vi "enablePWM.vi"(7 "targetTorque":i16, 8 "error in (no error)":errorcluster, 10 "targetVelocity":i32, 11 "MotorController in":refnum<class "MotorController.lvclass">) -> (0 "error out":errorcluster, 3 "MotorController out":refnum<class "MotorController.lvclass">)   [LabVIEW 2017, in "MotorController.lvclass"]
uses:
  MotorController.lvclass
  <vilib>/CANopenLib/CANOPEN.llb/CANopen Convert To Data [U16].vi
  <vilib>/CANopenLib/CANOPEN.llb/CANopen Convert To Data [I32].vi
  <vilib>/CANopenLib/CANOPEN.llb/CANopen Convert To Data [I16].vi
panel:
  in  "PDOChannel":u8(ring) items=["PDO 1", "PDO 2", "PDO 3", "PDO 4"]
  in  "CANopen data in":u8[](array[numeric])=[0, 0, 0, 0, 0, 0, 0, 0] format="%.0x"
  out "interface object out":refnum<k20>
  in  "interface object in":refnum<k20>
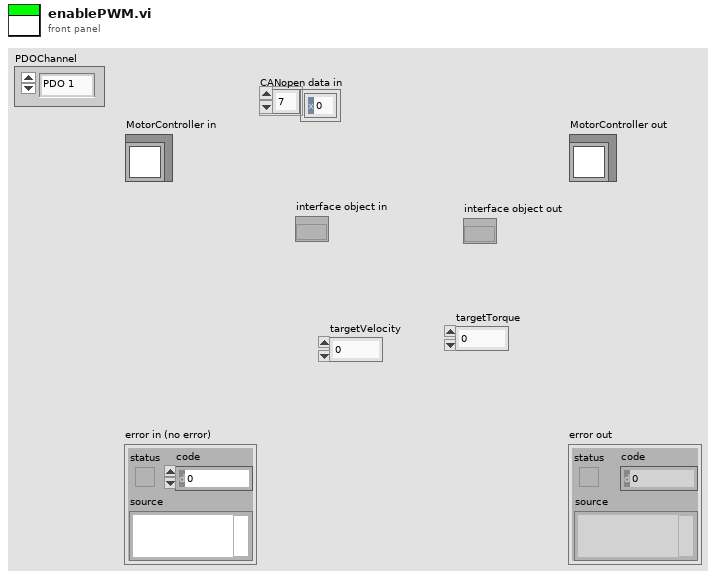
[diagram p1: front panel]
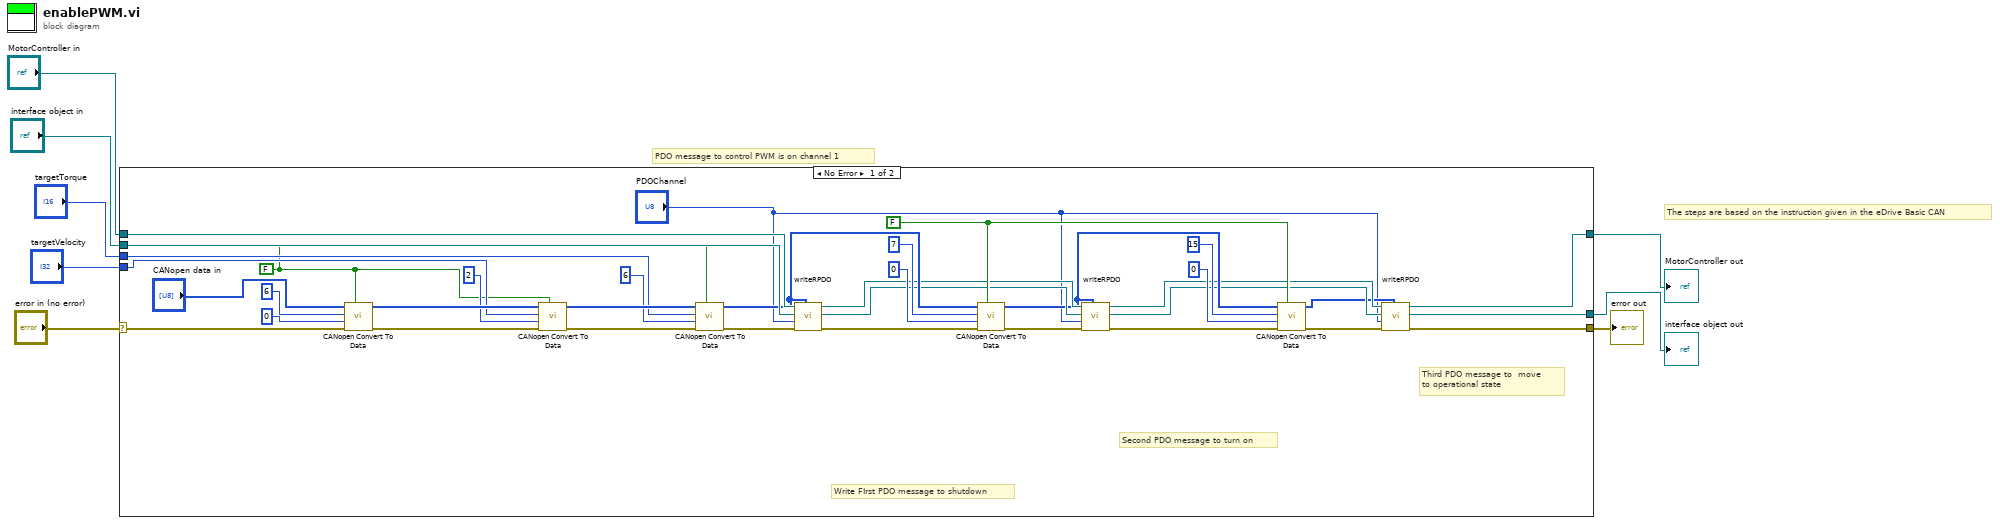
[diagram p0: block diagram]
diagram:
  # "The steps are based on the instruction given in the eDrive Basic CAN"
  # "PDO message to control PWM is on channel 1"
  n1 = case shown="No Error" "error in (no error)" {
    selector: "error in (no error)" -> [w40 w47]
    tunnel: [w10 w47] -> w7
    tunnel: [w11 w46] -> w5
    tunnel: "MotorController in" -> [w44 w46]
    tunnel: "interface object in" -> [w43 w45]
    tunnel: "targetTorque" -> [w32 _]
    tunnel: "targetVelocity" -> [w36 _]
    tunnel: [w12 w45] -> w1
    frame No Error {
      w25 = FALSE ("trim")
      w30 = FALSE ("trim")
      # "Third PDO message to  move \nto operational state"
      # "Second PDO message to turn on"
      # "Write FIrst PDO message to shutdown"
      n2 = call-poly <vilib>:"CANopen Convert To Data.vi"("trim"=w30, "error in (no error)"=w40, "offset (0)"=u32 0, "unsigned 16-bit integer"=u16 6 ("element"), "CANopen data in"="CANopen data in") -> ("error out"=w38:errorcluster, "CANopen data out"=w37:u8[])  [unwired: 5 in]
      n3 = call-poly <vilib>:"CANopen Convert To Data.vi"("trim"=w30, "error in (no error)"=w38, "offset (0)"=u32 2, "signed 32-bit integer"=w36, "CANopen data in"=w37) -> ("error out"=w34:errorcluster, "CANopen data out"=w33:u8[])  [unwired: 5 in]
      n4 = call-poly <vilib>:"CANopen Convert To Data.vi"("trim"=w30, "error in (no error)"=w34, "offset (0)"=u32 6, "signed 16-bit integer"=w32, "CANopen data in"=w33) -> ("error out"=w29:errorcluster, "CANopen data out"=w24:u8[])  [unwired: 5 in]
      n5 = call "writeRPDO.vi"("RPDO data"=w24, "error in (no error)"=w29, "PDOChannel"="PDOChannel", "interface object in"=w43, "MotorController in"=w44) -> ("error out"=w23:errorcluster, "interface object out"=w21:refnum<k20>, "MotorController out"=w22:refnum<class "MotorController.lvclass">)  [unwired: 4 in]
      n6 = call-poly <vilib>:"CANopen Convert To Data.vi"("trim"=w25, "error in (no error)"=w23, "offset (0)"=u32 0, "unsigned 16-bit integer"=u16 7 ("element"), "CANopen data in"=w24) -> ("error out"=w20:errorcluster, "CANopen data out"=w17:u8[])  [unwired: 5 in]
      n7 = call "writeRPDO.vi"("RPDO data"=w17, "error in (no error)"=w20, "PDOChannel"="PDOChannel", "interface object in"=w21, "MotorController in"=w22) -> ("error out"=w19:errorcluster, "interface object out"=w16:refnum<k20>, "MotorController out"=w15:refnum<class "MotorController.lvclass">)  [unwired: 4 in]
      n8 = call-poly <vilib>:"CANopen Convert To Data.vi"("trim"=w25, "error in (no error)"=w19, "offset (0)"=u32 0, "unsigned 16-bit integer"=u16 15 ("element"), "CANopen data in"=w17) -> ("error out"=w14:errorcluster, "CANopen data out"=w13:u8[])  [unwired: 5 in]
      n9 = call "writeRPDO.vi"("RPDO data"=w13, "error in (no error)"=w14, "PDOChannel"="PDOChannel", "interface object in"=w16, "MotorController in"=w15) -> ("error out"=w10:errorcluster, "interface object out"=w12:refnum<k20>, "MotorController out"=w11:refnum<class "MotorController.lvclass">)  [unwired: 4 in]
    }
    frame Error {
    }
  }
  "error out" <- w7
  "MotorController out" <- w5
  "interface object out" <- w1
